vi "PR_UDP_Labview_Demo.vi"() -> ()   [LabVIEW 2017]
uses:
  D:/Projects/GUI/Power Rider Wrapper/PowerRiderDLLWrapper.dll
  PowerRiderDLLWrapper.dll
panel:
  in  "Port":u16=8030
  in  "address IP":string="192.168.1.50"
  in  "String":string
  in  "TripType Enum":T1(ring)
  in  "Status Enum":enum16{"OFF", "ON", "ERROR", "FOREVER OFF"}(ring)
  in  "address":u16=85
  in  "Dst add":u16=16
  out "CommIcon":bool
  # "Power Rider Demo"
  # "UDP interface"
  # "ver 1.0"
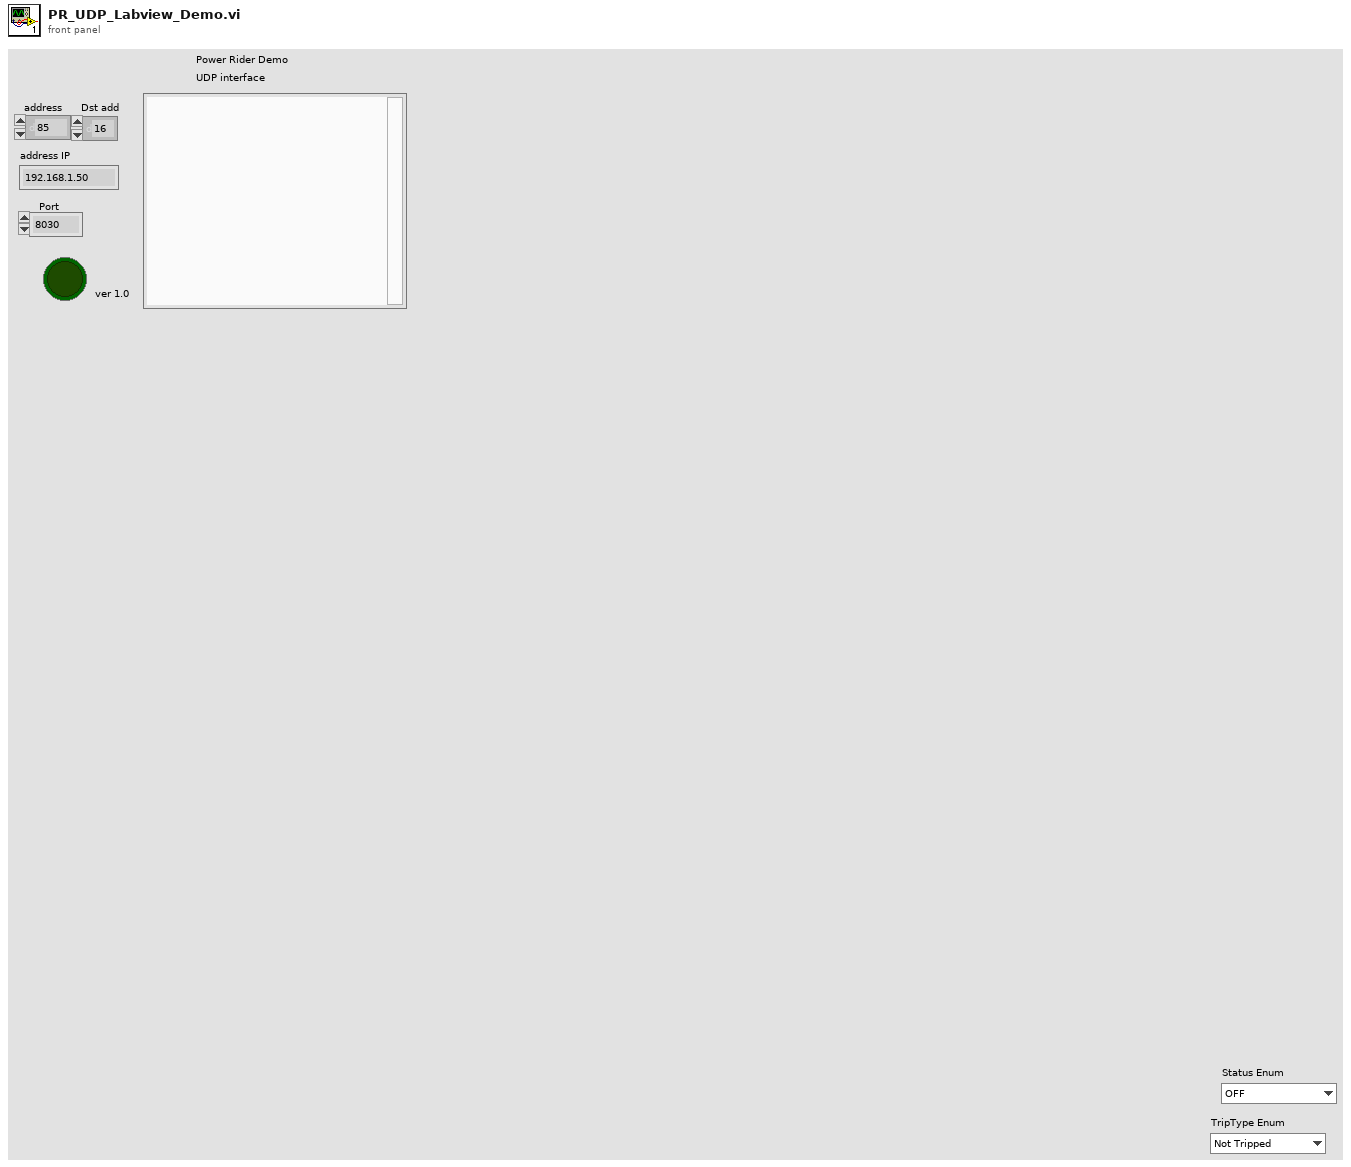
[diagram p1: front panel]
types:
  T1 = enum16{"Not Tripped", "SW Tripped", "Hard Short", "MAX SW Tripped"}
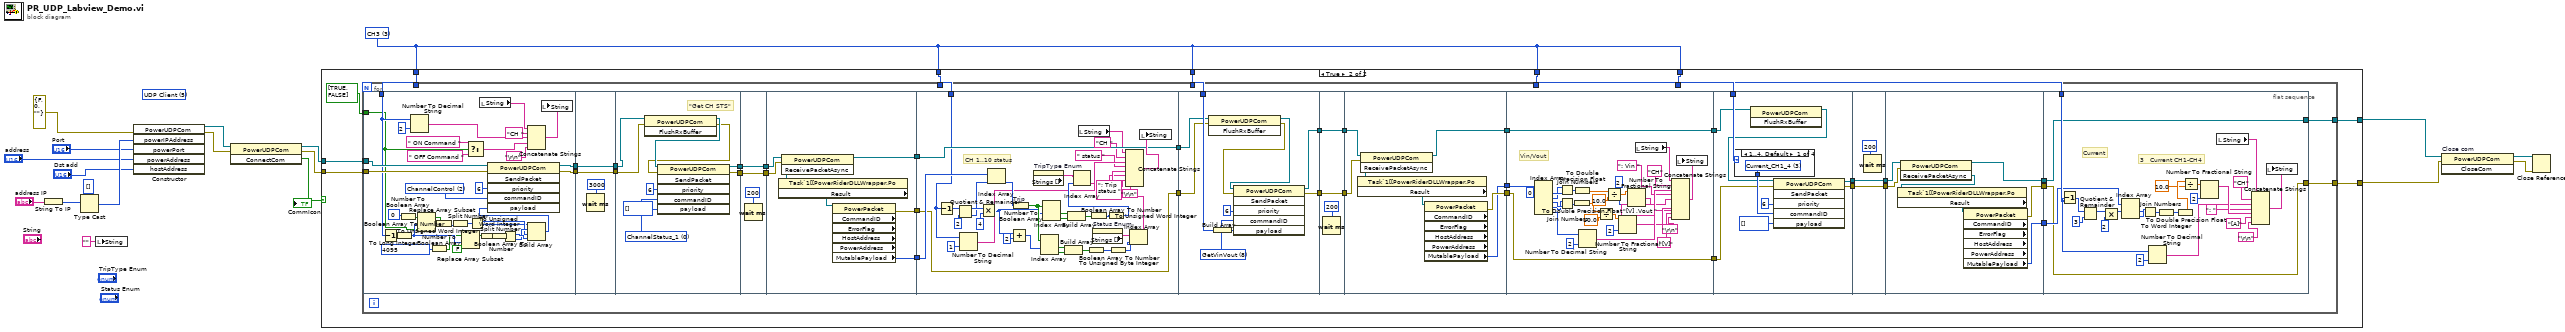
[diagram p0: block diagram]
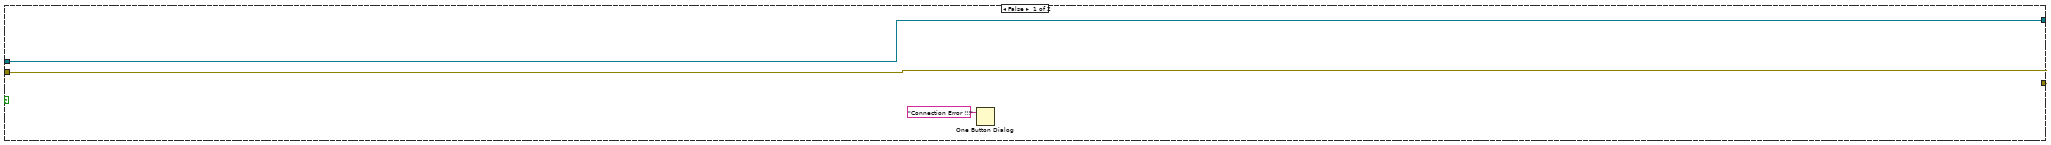
[diagram p2: hidden frame]
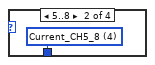
[diagram p3: hidden frame]
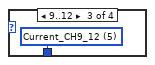
[diagram p4: hidden frame]
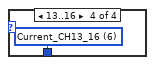
[diagram p5: hidden frame]
diagram:
  w4 = u8 3 items=["CH1"=1, "CH2"=2, "CH3"=3, "CH4"=4, "CH5"=5, "CH6"=6, "CH7"=7, "CH8"=8, "CH9"=9, "CH10"=10, "CH11"=11, "CH12"=12, "CH13"=13, "CH14"=14, "CH15"=15, "CH16"=16] ("Select CH #")
  (unwired) u16 5 items=["CANalystII"=2, "TCP Client"=3, "TCP Server"=4, "UDP Client"=5, "Serial COM"=6, "CAN Kvaser"=7] ("COMType 2")
  n1 = String To IP(1:"address IP") -> (0:w18:u32)
  n2 = Type Cast(type=u8[] [] ("powerIPAddress"), x=w18) -> (*(type *) &x=w19:u8[])
  n3 = local write "String"("" ("String")) -> ()
  n4 = constructor class="PowerUDPCom"(error in=errorcluster {"status"=FALSE, "code"=0, "source"=""} ("error out"), "powerIPAddress"=w19, "powerPort"="Port", "powerAddress"="address", "hostAddress"="Dst add") -> (reference out=w12:refnum<k24>, error out=w11:errorcluster)  [unwired: 2 in, 5 out]
  n5 = invoke class="PowerUDPCom" method="ConnectCom"(reference=w12, error in=w11) -> (reference out=w8:refnum<k24>, error out=w7:errorcluster, "ConnectCom"=w9:bool)  [unwired: 1 in]
  "CommIcon" <- w9
  n6 = case shown="True" w9 {
    tunnel: w8 -> [w21 w27]
    tunnel: w7 -> [w22 w26]
    tunnel: w4 -> [_ w32]
    tunnel: w4 -> [_ w31]
    tunnel: w4 -> [_ w30]
    tunnel: w4 -> [_ w29]
    tunnel: w4 -> [_ w28]
    tunnel: [w21 w25] -> w3
    tunnel: [w22 w24] -> w2
    frame False {
      n7 = One Button Dialog(message="Connection Error !!!") -> ()  [unwired: 1 in, 1 out]
    }
    frame True {
      n8 = for {
        tunnel: w32 -> [w60]
        tunnel: w31 -> [w59]
        tunnel: w30 -> [w58]
        tunnel: w29 -> [w57]
        tunnel: w28 -> [w56]
        tunnel: w27 -> [w55]
        tunnel: w26 -> [w54]
        tunnel: [w53] -> w25
        tunnel: [w52] -> w24
        tunnel: bool[] [TRUE, FALSE] -> [w51] mode=indexing
        n9 = flat-sequence {
          tunnel: w54 -> [w85]
          tunnel: [w87] -> w71
          tunnel: [w86] -> w70
          tunnel: w56 -> [w80]
          tunnel: w55 -> [w84]
          tunnel: w51 -> [w76]
          tunnel: w71 -> [w109]
          tunnel: [w109] -> w69
          tunnel: w70 -> [w108]
          tunnel: [w108] -> w68
          tunnel: [w115] -> w50
          tunnel: [w114] -> w48
          tunnel: w69 -> [w113]
          tunnel: w68 -> [w112]
          tunnel: w50 -> [w121]
          tunnel: [w121] -> w49
          tunnel: w48 -> [w120]
          tunnel: [w120] -> w47
          tunnel: w49 -> [w125]
          tunnel: w47 -> [w126]
          tunnel: [w124] -> w67
          tunnel: [w123] -> w66
          tunnel: [w122] -> w65
          tunnel: w67 -> [w134]
          tunnel: w66 -> [w137]
          tunnel: w65 -> [w135]
          tunnel: [w135] -> w64
          tunnel: [w134] -> w63
          tunnel: w60 -> [w132]
          tunnel: w64 -> [w168]
          tunnel: w63 -> [w166]
          tunnel: w59 -> [w169]
          tunnel: [w171] -> w46
          tunnel: [w170] -> w45
          tunnel: w46 -> [w177]
          tunnel: [w177] -> w43
          tunnel: w45 -> [w176]
          tunnel: [w176] -> w41
          tunnel: [w178] -> w44
          tunnel: w43 -> [w182]
          tunnel: [w180] -> w42
          tunnel: w41 -> [w181]
          tunnel: [w179] -> w40
          tunnel: w44 -> [w190]
          tunnel: [w186] -> w62
          tunnel: w42 -> [w186]
          tunnel: w40 -> [w185]
          tunnel: [w185] -> w61
          tunnel: w58 -> [w222]
          tunnel: w62 -> [w216]
          tunnel: w61 -> [w221]
          tunnel: [w218] -> w39
          tunnel: [w217] -> w38
          tunnel: w39 -> [w230]
          tunnel: [w230] -> w37
          tunnel: w38 -> [w229]
          tunnel: [w229] -> w35
          tunnel: w37 -> [w235]
          tunnel: [w232] -> w36
          tunnel: w35 -> [w236]
          tunnel: [w234] -> w34
          tunnel: [w233] -> w33
          tunnel: w36 -> [w238]
          tunnel: w34 -> [w239]
          tunnel: w57 -> [w244]
          tunnel: w33 -> [w243]
          tunnel: [w239] -> w53
          tunnel: [w238] -> w52
          frame #0 {
            w88 = u8 2 items=["ChannelStatus_1"=0, "ChannelControl"=2, "Current_CH1_4"=3, "Current_CH5_8"=4, "Current_CH9_12"=5, "Current_CH13_16"=6, "GetVinVout"=8, "Version_BoardType"=9, "SystemTemp"=10, "SystemParameter"=11, "ChannelParameter"=12, "GetTripEvent"=15, "LogFile"=18, "Configuration"=19, "ProductionData"=20, "BIT"=33, "DiscretePorts"=34, "SerialNumber"=36, "OffsetMeasurement"=37, "PartNumber"=39, "ChannelCombinedStatus_1_CH1_8"=40, "ChannelCombinedStatus_2_CH9_12"=41, "PlotData"=45, "PlotCommand"=46, "InternalData"=47, "KeepAlive"=234, "WakeUp"=250] ("commandID")
            n10 = Decrement(x=w80) -> (x-1=w89:u8)
            n11 = To Long Integer(number=w89) -> (32bit integer=w95:i32)
            n12 = Number To Boolean Array(number=u16 0 ("element")) -> (Boolean array=w91:bool[])
            n13 = Number To Decimal String(number=w80, width (-)=i16 2) -> (decimal integer string=w77:string)
            n14 = Replace Array Subset(array=w91, new element=w76, index=w95) -> (w92:bool[])
            n15 = Number To Boolean Array(number=u16 4095 ("mask")) -> (Boolean array=w94:bool[])
            n16 = Boolean Array To Number(Boolean array=w92) -> (number=w93:u32)
            n17 = To Unsigned Word Integer(number=w93) -> (unsigned 16bit integer=w100:u16)
            n18 = Replace Array Subset(array=w94, new element=FALSE ("new element/subarray"), index=w95) -> (w90:bool[])
            n19 = Select(t=" ON Command " ("string"), s=w76, f=" OFF Command " ("string")) -> (s? t:f=w73:string)
            n20 = Split Number(x=w100) -> (hi(x)=w104:u8, lo(x)=w103:u8)
            n21 = local read "String"() -> (w82:string)
            n22 = Boolean Array To Number(Boolean array=w90) -> (number=w99:u32)
            n23 = To Unsigned Word Integer(number=w99) -> (unsigned 16bit integer=w102:u16)
            n24 = Split Number(x=w102) -> (hi(x)=w106:u8, lo(x)=w105:u8)
            n25 = Concatenate Strings(w82, "CH " ("string"), w77, w73, "\r\n") -> (w81:string)
            n26 = Build Array(w103, w105, w104, w106) -> (w101:u8[])
            n27 = invoke class="PowerUDPCom" method="SendPacket"(reference=w84, error in=w85, "priority"=u8 6, "commandID"=w88, "payload"=w101) -> (reference out=w87:refnum<k24>, error out=w86:errorcluster)  [unwired: 1 in, 4 out]
            n28 = local write "String"(w81) -> ()
          }
          frame #1 {
            n29 = Wait (ms)(milliseconds to wait=u32 3000) -> ()  [unwired: 1 out]
          }
          frame #2 {
            w118 = u8 0 items=["ChannelStatus_1"=0, "ChannelControl"=2, "Current_CH1_4"=3, "Current_CH5_8"=4, "Current_CH9_12"=5, "Current_CH13_16"=6, "GetVinVout"=8, "Version_BoardType"=9, "SystemTemp"=10, "SystemParameter"=11, "ChannelParameter"=12, "GetTripEvent"=15, "LogFile"=18, "Configuration"=19, "ProductionData"=20, "BIT"=33, "DiscretePorts"=34, "SerialNumber"=36, "OffsetMeasurement"=37, "PartNumber"=39, "ChannelCombinedStatus_1_CH1_8"=40, "ChannelCombinedStatus_2_CH9_12"=41, "PlotData"=45, "PlotCommand"=46, "InternalData"=47, "KeepAlive"=234, "WakeUp"=250] ("commandID")
            # "\"Get CH STS\""
            n30 = invoke class="PowerUDPCom" method="FlushRxBuffer"(reference=w113, error in=w112) -> (reference out=w111:refnum<k24>, error out=w110:errorcluster)  [unwired: 1 in, 1 out]
            n31 = invoke class="PowerUDPCom" method="SendPacket"(reference=w111, error in=w110, "priority"=u8 6, "commandID"=w118, "payload"=u8[] []) -> (reference out=w114:refnum<k24>, error out=w115:errorcluster)  [unwired: 1 in, 4 out]
          }
          frame #3 {
            n32 = Wait (ms)(milliseconds to wait=u32 200) -> ()  [unwired: 1 out]
          }
          frame #4 {
            n33 = invoke class="PowerUDPCom" method="ReceivePacketAsync"(reference=w126, error in=w125) -> (reference out=w122:refnum<k24>, "ReceivePacketAsync"=w128:refnum<k24>)  [unwired: 1 in, 1 out]
            n34 = property class="Task`1[[PowerRiderDLLWrapper.Po"(reference=w128) -> ("Result"=w127:refnum<k24>)  [unwired: 1 in, 2 out]
            n35 = property class="PowerPacket" props=["CommandID", "ErrorFlag", "HostAddress", "PowerAddress", "MutablePayload"](reference=w127) -> (error out=w124:errorcluster, "MutablePayload"=w123:u8[])  [unwired: 1 in, 5 out]
          }
          frame #5 {
            # "CH 1..10 status"
            n36 = Decrement(x=w132) -> (x-1=w129:u8)
            n37 = Quotient & Remainder(x=w129, y=2) -> (x-y*floor(x/y)=w147:i32, floor(x/y)=w146:i32)
            n38 = Number To Decimal String(number=w132, width (-)=i16 1) -> (decimal integer string=w150:string)
            n39 = Multiply(x=w147, y=u8 4) -> (x*y=w145:i32)
            n40 = Index Array(array=w137, index=w146) -> (element=w152:u8)
            n41 = Add(x=w145, y=u8 2) -> (x+y=w144:i32)
            n42 = Number To Boolean Array "Trip"(number=w152) -> (Boolean array=w151:bool[])
            n43 = property on="TripType Enum" class="Enum (strict)"() -> ("Strings []"=w161:string[])  [unwired: 2 in, 2 out]
            n44 = Index Array(array=w151, index #1=w144) -> (element #1=w160:bool, element #2=w159:bool)  [unwired: 1 in]
            n45 = Index Array(array=w151, index #1=w145) -> (element #1=w157:bool, element #2=w158:bool)  [unwired: 1 in]
            n46 = Build Array(w160, w159) -> (w156:bool[])
            n47 = Build Array(w157, w158) -> (w155:bool[])
            n48 = local read "String"() -> (w131:string)
            n49 = Boolean Array To Number(Boolean array=w156) -> (number=w154:u32)
            n50 = Boolean Array To Number(Boolean array=w155) -> (number=w153:u32)
            n51 = property on="Status Enum" class="Enum (strict)"() -> ("Strings []"=w162:string[])  [unwired: 2 in, 2 out]
            n52 = To Unsigned Word Integer(number=w153) -> (unsigned 16bit integer=w163:u16)
            n53 = Index Array(array=w161, index=w163) -> (element=w149:string)
            n54 = To Unsigned Byte Integer(number=w154) -> (unsigned 8bit integer=w164:u8)
            n55 = Index Array(array=w162, index=w164) -> (element=w148:string)
            n56 = Concatenate Strings(w131, "CH " ("string"), w150, " status ", w148, "; Trip status ", w149, "\r\n") -> (w136:string)
            n57 = local write "String"(w136) -> ()
          }
          frame #6 {
            w173 = u8 8 items=["ChannelStatus_1"=0, "ChannelControl"=2, "Current_CH1_4"=3, "Current_CH5_8"=4, "Current_CH9_12"=5, "Current_CH13_16"=6, "GetVinVout"=8, "Version_BoardType"=9, "SystemTemp"=10, "SystemParameter"=11, "ChannelParameter"=12, "GetTripEvent"=15, "LogFile"=18, "Configuration"=19, "ProductionData"=20, "BIT"=33, "DiscretePorts"=34, "SerialNumber"=36, "OffsetMeasurement"=37, "PartNumber"=39, "ChannelCombinedStatus_1_CH1_8"=40, "ChannelCombinedStatus_2_CH9_12"=41, "PlotData"=45, "PlotCommand"=46, "InternalData"=47, "KeepAlive"=234, "WakeUp"=250] ("commandID")
            n58 = invoke class="PowerUDPCom" method="FlushRxBuffer"(reference=w168, error in=w166) -> (reference out=w167:refnum<k24>, error out=w165:errorcluster)  [unwired: 1 in, 1 out]
            n59 = Build Array(w169) -> (w174:u8[])
            n60 = invoke class="PowerUDPCom" method="SendPacket"(reference=w167, error in=w165, "priority"=u8 6, "commandID"=w173, "payload"=w174) -> (reference out=w171:refnum<k24>, error out=w170:errorcluster)  [unwired: 1 in, 4 out]
          }
          frame #7 {
            n61 = Wait (ms)(milliseconds to wait=u32 200) -> ()  [unwired: 1 out]
          }
          frame #8 {
            n62 = invoke class="PowerUDPCom" method="ReceivePacketAsync"(reference=w182, error in=w181) -> (reference out=w180:refnum<k24>, "ReceivePacketAsync"=w184:refnum<k24>)  [unwired: 1 in, 1 out]
            n63 = property class="Task`1[[PowerRiderDLLWrapper.Po"(reference=w184) -> ("Result"=w183:refnum<k24>)  [unwired: 1 in, 2 out]
            n64 = property class="PowerPacket" props=["CommandID", "ErrorFlag", "HostAddress", "PowerAddress", "MutablePayload"](reference=w183) -> (error out=w179:errorcluster, "MutablePayload"=w178:u8[])  [unwired: 1 in, 5 out]
          }
          frame #9 {
            # "Vin/Vout"
            n65 = Index Array(array=w190, index #1=0 ("index")) -> (element #1=w212:u8, element #2=w211:u8, element #3=w210:u8, element #4=w209:u8, element #5=w206:u8)  [unwired: 4 in]
            n66 = Join Numbers(hi=w211, lo=w212) -> ((hi.lo)=w213:u16)
            n67 = Join Numbers(hi=w209, lo=w210) -> ((hi.lo)=w214:u16)
            n68 = To Double Precision Float(number=w214) -> (double precision float=w207:dbl)
            n69 = To Double Precision Float(number=w213) -> (double precision float=w208:dbl)
            n70 = Number To Decimal String(number=w206, width (-)=i16 2) -> (decimal integer string=w205:string)
            n71 = Divide(x=w207, y=10.0) -> (x/y=w202:dbl)
            n72 = Divide(x=w208, y=10.0) -> (x/y=w204:dbl)
            n73 = Number To Fractional String(number=w202, precision (6)=i16 2) -> (F-format string=w201:string)  [unwired: 2 in]
            n74 = Number To Fractional String(number=w204, precision (6)=i16 2) -> (F-format string=w203:string)  [unwired: 2 in]
            n75 = local read "String"() -> (w188:string)
            n76 = Concatenate Strings(w188, "CH" ("string"), w205, ": Vin " ("string"), w203, "[V] ,Vout " ("string"), w201, "[V]" ("string"), "\r\n") -> (w189:string)
            n77 = local write "String"(w189) -> ()
          }
          frame #10 {
            n78 = case shown="1..4, Default" w222 {
              tunnel: [w224 w225 w226 w227] -> w223
              frame 1..4, Default {
                w224 = u8 3 items=["ChannelStatus_1"=0, "ChannelControl"=2, "Current_CH1_4"=3, "Current_CH5_8"=4, "Current_CH9_12"=5, "Current_CH13_16"=6, "GetVinVout"=8, "Version_BoardType"=9, "SystemTemp"=10, "SystemParameter"=11, "ChannelParameter"=12, "GetTripEvent"=15, "LogFile"=18, "Configuration"=19, "ProductionData"=20, "BIT"=33, "DiscretePorts"=34, "SerialNumber"=36, "OffsetMeasurement"=37, "PartNumber"=39, "ChannelCombinedStatus_1_CH1_8"=40, "ChannelCombinedStatus_2_CH9_12"=41, "PlotData"=45, "PlotCommand"=46, "InternalData"=47, "KeepAlive"=234, "WakeUp"=250] ("commandID")
              }
              frame 5..8 {
                w225 = u8 4 items=["ChannelStatus_1"=0, "ChannelControl"=2, "Current_CH1_4"=3, "Current_CH5_8"=4, "Current_CH9_12"=5, "Current_CH13_16"=6, "GetVinVout"=8, "Version_BoardType"=9, "SystemTemp"=10, "SystemParameter"=11, "ChannelParameter"=12, "GetTripEvent"=15, "LogFile"=18, "Configuration"=19, "ProductionData"=20, "BIT"=33, "DiscretePorts"=34, "SerialNumber"=36, "OffsetMeasurement"=37, "PartNumber"=39, "ChannelCombinedStatus_1_CH1_8"=40, "ChannelCombinedStatus_2_CH9_12"=41, "PlotData"=45, "PlotCommand"=46, "InternalData"=47, "KeepAlive"=234, "WakeUp"=250] ("commandID")
              }
              frame 9..12 {
                w226 = u8 5 items=["ChannelStatus_1"=0, "ChannelControl"=2, "Current_CH1_4"=3, "Current_CH5_8"=4, "Current_CH9_12"=5, "Current_CH13_16"=6, "GetVinVout"=8, "Version_BoardType"=9, "SystemTemp"=10, "SystemParameter"=11, "ChannelParameter"=12, "GetTripEvent"=15, "LogFile"=18, "Configuration"=19, "ProductionData"=20, "BIT"=33, "DiscretePorts"=34, "SerialNumber"=36, "OffsetMeasurement"=37, "PartNumber"=39, "ChannelCombinedStatus_1_CH1_8"=40, "ChannelCombinedStatus_2_CH9_12"=41, "PlotData"=45, "PlotCommand"=46, "InternalData"=47, "KeepAlive"=234, "WakeUp"=250] ("commandID")
              }
              frame 13..16 {
                w227 = u8 6 items=["ChannelStatus_1"=0, "ChannelControl"=2, "Current_CH1_4"=3, "Current_CH5_8"=4, "Current_CH9_12"=5, "Current_CH13_16"=6, "GetVinVout"=8, "Version_BoardType"=9, "SystemTemp"=10, "SystemParameter"=11, "ChannelParameter"=12, "GetTripEvent"=15, "LogFile"=18, "Configuration"=19, "ProductionData"=20, "BIT"=33, "DiscretePorts"=34, "SerialNumber"=36, "OffsetMeasurement"=37, "PartNumber"=39, "ChannelCombinedStatus_1_CH1_8"=40, "ChannelCombinedStatus_2_CH9_12"=41, "PlotData"=45, "PlotCommand"=46, "InternalData"=47, "KeepAlive"=234, "WakeUp"=250] ("commandID")
              }
            }
            n79 = invoke class="PowerUDPCom" method="FlushRxBuffer"(reference=w216) -> (reference out=w215:refnum<k24>)  [unwired: 2 in, 2 out]
            n80 = invoke class="PowerUDPCom" method="SendPacket"(reference=w215, error in=w221, "priority"=u8 6, "commandID"=w223, "payload"=u8[] []) -> (reference out=w217:refnum<k24>, error out=w218:errorcluster)  [unwired: 1 in, 4 out]
          }
          frame #11 {
            n81 = Wait (ms)(milliseconds to wait=u32 200) -> ()  [unwired: 1 out]
          }
          frame #12 {
            n82 = invoke class="PowerUDPCom" method="ReceivePacketAsync"(reference=w236, error in=w235) -> (reference out=w234:refnum<k24>, "ReceivePacketAsync"=w231:refnum<k24>)  [unwired: 1 in, 1 out]
            n83 = property class="Task`1[[PowerRiderDLLWrapper.Po"(reference=w231) -> ("Result"=w237:refnum<k24>)  [unwired: 1 in, 2 out]
            n84 = property class="PowerPacket" props=["CommandID", "ErrorFlag", "HostAddress", "PowerAddress", "MutablePayload"](reference=w237) -> (error out=w232:errorcluster, "MutablePayload"=w233:u8[])  [unwired: 1 in, 5 out]
          }
          frame #13 {
            # "3   Current CH1-CH4"
            # "Current"
            n85 = Decrement(x=w244) -> (x-1=w245:u8)
            n86 = Quotient & Remainder(x=w245, y=u8 3) -> (x-y*floor(x/y)=w259:u8)  [unwired: 1 out]
            n87 = Multiply(x=w259, y=u8 2) -> (x*y=w258:u8)
            n88 = Index Array(array=w243, index #1=w258) -> (element #1=w256:u8, element #2=w257:u8)  [unwired: 1 in]
            n89 = Join Numbers(hi=w257, lo=w256) -> ((hi.lo)=w260:u16)
            n90 = Number To Decimal String(number=w244, width (-)=i16 2) -> (decimal integer string=w254:string)
            n91 = To Word Integer(number=w260) -> (16bit integer=w262:i16)
            n92 = To Double Precision Float(number=w262) -> (double precision float=w261:dbl)
            n93 = Divide(x=w261, y=10.0) -> (x/y=w255:dbl)
            n94 = Number To Fractional String(number=w255, precision (6)=i16 2) -> (F-format string=w263:string)  [unwired: 2 in]
            n95 = local read "String"() -> (w240:string)
            n96 = Concatenate Strings(w240, "CH" ("string"), w254, ": " ("string"), w263, "[A]" ("string"), "\r\n") -> (w242:string)
            n97 = local write "String"(w242) -> ()
          }
        }
      }
    }
  }
  n98 = invoke on="Close com" class="PowerUDPCom" method="CloseCom"(reference=w3, error in=w2) -> (reference out=w6:refnum<k24>, error out=w5:errorcluster)  [unwired: 1 in, 1 out]
  n99 = Close Reference(reference=w6, error in (no error)=w5) -> ()  [unwired: 1 out]
